vi "TwH5ErrorConvert.vi"(8 "error in (no error)":errorcluster, 11 "error code":i32) -> (0 "error out":errorcluster)   [LabVIEW 2009]
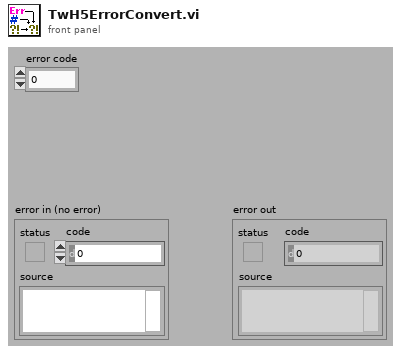
[diagram p1: front panel]
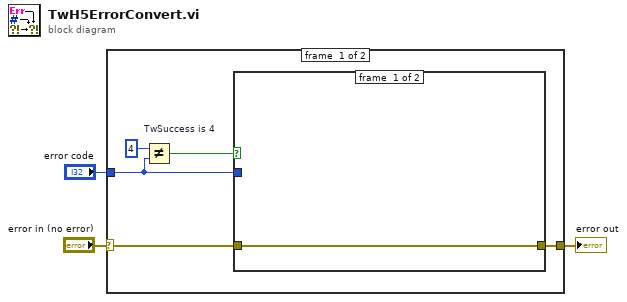
[diagram p0: block diagram]
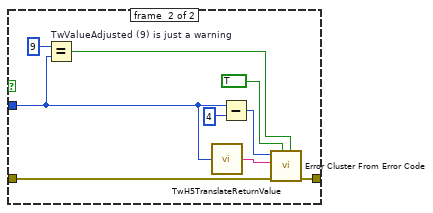
[diagram p2: hidden frame]
diagram:
  n1 = case shown="No Error" "error in (no error)" {
    selector: "error in (no error)" -> [w7 w19]
    tunnel: [w5 w19] -> w2
    tunnel: "error code" -> [w6 _]
    frame #0 {
      n2 = Not Equal? "TwSuccess is 4"(x=4, y=w6) -> (x != y?=w8:bool)
      n3 = case shown="True" w8 {
        tunnel: w7 -> [w9 w18]
        tunnel: w6 -> [_ w10]
        tunnel: [w9 w17] -> w5
        frame #0 {
        }
        frame #1 {
          n4 = Equal? "TwValueAdjusted (9) is just a warning"(x=9, y=w10) -> (x = y?=w12:bool)
          n5 = call "TwH5TranslateReturnValue.vi"("TwRetVal"=w10) -> ("return type"=w15:string)
          n6 = Subtract(x=w10, y=4 ("x")) -> (x-y=w14:i32)
          n7 = call <vilib>:"Error Cluster From Error Code.vi"("is warning? (False)"=w12, "show call chain? (False)"=TRUE, "error in (no error)"=w18, "error message (\"\")"=w15, "error code (0)"=w14) -> ("error out"=w17:errorcluster)  [unwired: 4 out]
        }
      }
    }
    frame #1 {
    }
  }
  "error out" <- w2
